vi "E2E Call VI.vi"() -> ()   [LabVIEW 2020]
panel:
  out "Control Value:Get 4":variant
  out "Control Value:Get 3":variant
  out "Control Value:Get 2":variant
  out "Control Value:Get":variant
  out "Control Value:Get All":cluster{"Name":string, "Variant Data":variant}[](array[cluster])
  out "error out":errorcluster
  in  "vi path":path
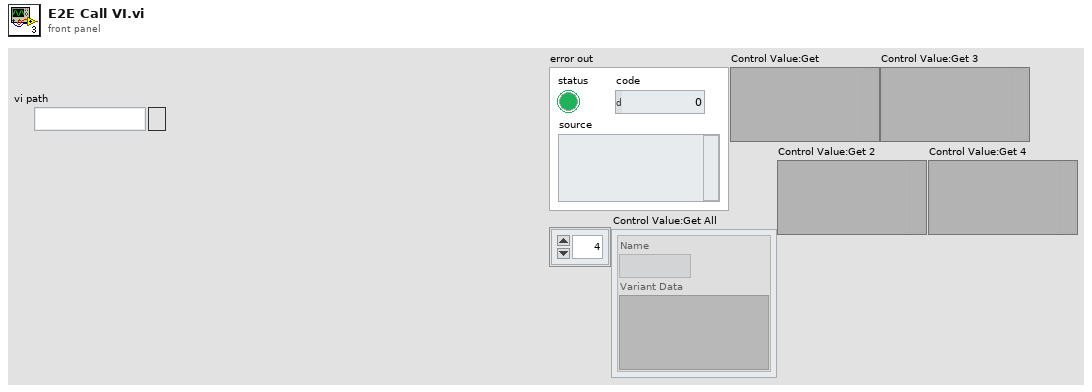
[diagram p1: front panel]
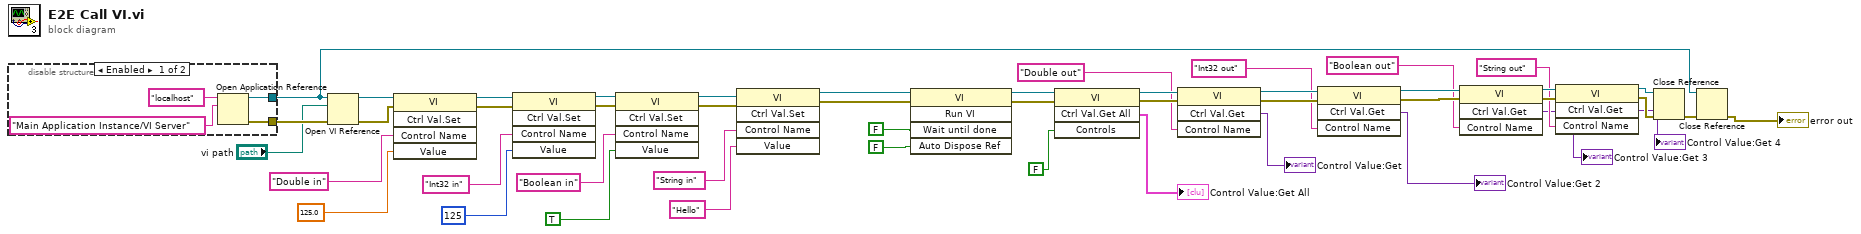
[diagram p0: block diagram]
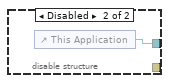
[diagram p2: hidden frame]
diagram:
  n1 = disable-structure shown="Enabled" {
    disable-tunnel: [w51 _] -> w47
    disable-tunnel: [w50 w52] -> w45
    frame Enabled {
      n2 = Open Application Reference(10:"Main Application Instance/VI Server" ("machine name (\"\":  open local reference)"), 11:"localhost" ("machine name (\"\":  open local reference)")) -> (0:w51:errorcluster, 3:w50:refnum<vi>)  [unwired: 2 in]
    }
    frame Disabled {
      n3 = control-ref of="This Application"() -> (w52:refnum<vi>)
    }
  }
  n4 = Open VI Reference(application reference (local)=w45, vi path="vi path", error in (no error)=w47) -> (vi reference=w44:refnum<vi>, error out=w38:errorcluster)  [unwired: 3 in]
  n5 = invoke class="VI" method="Ctrl Val.Set"(reference=w44, error in=w38, "Control Name"="Double in", "Value"=125.0) -> (reference out=w33:refnum<vi>, error out=w32:errorcluster)  [unwired: 1 in, 3 out]
  n6 = invoke class="VI" method="Ctrl Val.Set"(reference=w33, error in=w32, "Control Name"="Int32 in", "Value"=125) -> (reference out=w37:refnum<vi>, error out=w36:errorcluster)  [unwired: 1 in, 3 out]
  n7 = invoke class="VI" method="Ctrl Val.Set"(reference=w37, error in=w36, "Control Name"="Boolean in", "Value"=TRUE) -> (reference out=w35:refnum<vi>, error out=w34:errorcluster)  [unwired: 1 in, 3 out]
  n8 = invoke class="VI" method="Ctrl Val.Set"(reference=w35, error in=w34, "Control Name"="String in", "Value"="Hello" ("Control Name")) -> (reference out=w23:refnum<vi>, error out=w22:errorcluster)  [unwired: 1 in, 3 out]
  n9 = invoke class="VI" method="Run VI"(reference=w23, error in=w22, "Wait until done"=FALSE ("Wait Until Done"), "Auto Dispose Ref"=FALSE ("Auto Dispose Reference")) -> (reference out=w21:refnum<vi>, error out=w41:errorcluster)  [unwired: 1 in, 3 out]
  n10 = invoke class="VI" method="Ctrl Val.Get All"(reference=w21, error in=w41, "Controls"=FALSE) -> (reference out=w18:refnum<vi>, error out=w17:errorcluster, "Get All Control Values Variant"=→"Control Value:Get All":cluster{"Name":string, "Variant Data":variant}[])  [unwired: 1 in, 1 out]
  n11 = invoke class="VI" method="Ctrl Val.Get"(reference=w18, error in=w17, "Control Name"="Double out") -> (reference out=w12:refnum<vi>, error out=w11:errorcluster, "Get Control Value Variant"=→"Control Value:Get":variant)  [unwired: 1 in, 1 out]
  n12 = invoke class="VI" method="Ctrl Val.Get"(reference=w12, error in=w11, "Control Name"="Int32 out") -> (reference out=w10:refnum<vi>, error out=w9:errorcluster, "Get Control Value Variant"=→"Control Value:Get 2":variant)  [unwired: 1 in, 1 out]
  n13 = invoke class="VI" method="Ctrl Val.Get"(reference=w10, error in=w9, "Control Name"="Boolean out") -> (reference out=w16:refnum<vi>, error out=w15:errorcluster, "Get Control Value Variant"=→"Control Value:Get 3":variant)  [unwired: 1 in, 1 out]
  n14 = invoke class="VI" method="Ctrl Val.Get"(reference=w16, error in=w15, "Control Name"="String out") -> (reference out=w14:refnum<vi>, error out=w13:errorcluster, "Get Control Value Variant"=→"Control Value:Get 4":variant)  [unwired: 1 in, 1 out]
  n15 = Close Reference(reference=w14, error in (no error)=w13) -> (error out=w46:errorcluster)
  n16 = Close Reference(reference=w45, error in (no error)=w46) -> (error out=→"error out":errorcluster)
